vi "Write Functions.vi"(5 "Functions":variant=variant("Absolute Value"=variant(refnum<class "PythonFunction.lvclass"> refnum), "Add"=variant(refnum<class "PythonFunction.lvclass"> refnum), "And"=variant(refnum<class "PythonFunction.lvclass"> refnum), "And Array Elements"=variant(refnum<class "PythonFunction.lvclass"> refnum), "Array Max & Min"=variant(refnum<class "PythonFunction.lvclass"> refnum), "Array Size"=variant(refnum<class "PythonFunction.lvclass"> refnum), "Array Subset"=variant(refnum<class "PythonFunction.lvclass"> refnum), "Array of Strings To Path"=variant(refnum<class "PythonFunction.lvclass"> refnum), "Build Array"=variant(refnum<class "PythonFunction.lvclass"> refnum), "Build Path"=variant(refnum<class "PythonFunction.lvclass"> refnum), "Byte Array To String"=variant(refnum<class "PythonFunction.lvclass"> refnum), "Close File"=variant(refnum<class "PythonFunction.lvclass"> refnum), "Concatenate Strings"=variant(refnum<class "PythonFunction.lvclass"> refnum), "Cosecant"=variant(refnum<class "PythonFunction.lvclass"> refnum), "Cosine"=variant(refnum<class "PythonFunction.lvclass"> refnum), "Cotangent"=variant(refnum<class "PythonFunction.lvclass"> refnum), "Decimal String To Number"=variant(refnum<class "PythonFunction.lvclass"> refnum), "Decimate 1D Array"=variant(refnum<class "PythonFunction.lvclass"> refnum), "Delete From Array"=variant(refnum<class "PythonFunction.lvclass"> refnum), "Divide"=variant(refnum<class "PythonFunction.lvclass"> refnum), "Empty Array?"=variant(refnum<class "PythonFunction.lvclass"> refnum), "Empty String/Path?"=variant(refnum<class "PythonFunction.lvclass"> refnum), "Equal To 0?"=variant(refnum<class "PythonFunction.lvclass"> refnum), "Equal?"=variant(refnum<class "PythonFunction.lvclass"> refnum), "Exclusive Or"=variant(refnum<class "PythonFunction.lvclass"> refnum), "Exponential"=variant(refnum<class "PythonFunction.lvclass"> refnum), "Exponential(Arg)-1"=variant(refnum<class "PythonFunction.lvclass"> refnum), "Format Value"=variant(refnum<class "PythonFunction.lvclass"> refnum), "Fract/Exp String To Number"=variant(refnum<class "PythonFunction.lvclass"> refnum), "Get Date/Time String"=variant(refnum<class "PythonFunction.lvclass"> refnum), "Greater Or Equal To 0?"=variant(refnum<class "PythonFunction.lvclass"> refnum), "Greater Or Equal?"=variant(refnum<class "PythonFunction.lvclass"> refnum), "Greater Than 0?"=variant(refnum<class "PythonFunction.lvclass"> refnum), "Greater?"=variant(refnum<class "PythonFunction.lvclass"> refnum), "Hexadecimal String To Number"=variant(refnum<class "PythonFunction.lvclass"> refnum), "Hyperbolic Cosecant"=variant(refnum<class "PythonFunction.lvclass"> refnum), "Hyperbolic Cosine"=variant(refnum<class "PythonFunction.lvclass"> refnum), "Hyperbolic Cotangent"=variant(refnum<class "PythonFunction.lvclass"> refnum), "Hyperbolic Secant"=variant(refnum<class "PythonFunction.lvclass"> refnum), "Hyperbolic Sine"=variant(refnum<class "PythonFunction.lvclass"> refnum), "Hyperbolic Tangent"=variant(refnum<class "PythonFunction.lvclass"> refnum), "Implies"=variant(refnum<class "PythonFunction.lvclass"> refnum), "In Range and Coerce"=variant(refnum<class "PythonFunction.lvclass"> refnum), "Index Array"=variant(refnum<class "PythonFunction.lvclass"> refnum), "Initialize Array"=variant(refnum<class "PythonFunction.lvclass"> refnum), "Interleave 1D Arrays"=variant(refnum<class "PythonFunction.lvclass"> refnum), "Inverse Cosecant"=variant(refnum<class "PythonFunction.lvclass"> refnum), "Inverse Cosine"=variant(refnum<class "PythonFunction.lvclass"> refnum), "Inverse Cotangent"=variant(refnum<class "PythonFunction.lvclass"> refnum), "Inverse Hyperbolic Cosecant"=variant(refnum<class "PythonFunction.lvclass"> refnum), "Inverse Hyperbolic Cosine"=variant(refnum<class "PythonFunction.lvclass"> refnum), "Inverse Hyperbolic Cotangent"=variant(refnum<class "PythonFunction.lvclass"> refnum), "Inverse Hyperbolic Secant"=variant(refnum<class "PythonFunction.lvclass"> refnum), "Inverse Hyperbolic Sine"=variant(refnum<class "PythonFunction.lvclass"> refnum), "Inverse Hyperbolic Tangent"=variant(refnum<class "PythonFunction.lvclass"> refnum), "Inverse Secant"=variant(refnum<class "PythonFunction.lvclass"> refnum), "Inverse Sine"=variant(refnum<class "PythonFunction.lvclass"> refnum), "Inverse Tangent"=variant(refnum<class "PythonFunction.lvclass"> refnum), "Inverse Tangent (2 Input)"=variant(refnum<class "PythonFunction.lvclass"> refnum), "Less Or Equal To 0?"=variant(refnum<class "PythonFunction.lvclass"> refnum), "Less Or Equal?"=variant(refnum<class "PythonFunction.lvclass"> refnum), "Less Than 0?"=variant(refnum<class "PythonFunction.lvclass"> refnum), "Less?"=variant(refnum<class "PythonFunction.lvclass"> refnum), "Lexical Class"=variant(refnum<class "PythonFunction.lvclass"> refnum), "Logarithm Base 10"=variant(refnum<class "PythonFunction.lvclass"> refnum), "Logarithm Base 2"=variant(refnum<class "PythonFunction.lvclass"> refnum), "Max & Min"=variant(refnum<class "PythonFunction.lvclass"> refnum), "Multiply"=variant(refnum<class "PythonFunction.lvclass"> refnum), "Natural Logarithm"=variant(refnum<class "PythonFunction.lvclass"> refnum), "Negate"=variant(refnum<class "PythonFunction.lvclass"> refnum), "Not"=variant(refnum<class "PythonFunction.lvclass"> refnum), "Not A Number/Path/Refnum?"=variant(refnum<class "PythonFunction.lvclass"> refnum), "Not And"=variant(refnum<class "PythonFunction.lvclass"> refnum), "Not Equal To 0?"=variant(refnum<class "PythonFunction.lvclass"> refnum), "Not Equal?"=variant(refnum<class "PythonFunction.lvclass"> refnum), "Not Exclusive Or"=variant(refnum<class "PythonFunction.lvclass"> refnum), "Not Or"=variant(refnum<class "PythonFunction.lvclass"> refnum), "Number To Boolean Array"=variant(refnum<class "PythonFunction.lvclass"> refnum), "Number To Decimal String"=variant(refnum<class "PythonFunction.lvclass"> refnum), "Number To Exponential String"=variant(refnum<class "PythonFunction.lvclass"> refnum), "Number To Fractional String"=variant(refnum<class "PythonFunction.lvclass"> refnum), "Number To Hexadecimal String"=variant(refnum<class "PythonFunction.lvclass"> refnum), "Number To Octal String"=variant(refnum<class "PythonFunction.lvclass"> refnum), "Octal String To Number"=variant(refnum<class "PythonFunction.lvclass"> refnum), "Open/Create/Replace File"=variant(refnum<class "PythonFunction.lvclass"> refnum), "Or"=variant(refnum<class "PythonFunction.lvclass"> refnum), "Or Array Elements"=variant(refnum<class "PythonFunction.lvclass"> refnum), "Path To String"=variant(refnum<class "PythonFunction.lvclass"> refnum), "Path to Array of Strings"=variant(refnum<class "PythonFunction.lvclass"> refnum), "Power of 2"=variant(refnum<class "PythonFunction.lvclass"> refnum), "Power of X"=variant(refnum<class "PythonFunction.lvclass"> refnum), "Quotient & Remainder"=variant(refnum<class "PythonFunction.lvclass"> refnum), "Random Number (0-1)"=variant(refnum<class "PythonFunction.lvclass"> refnum), "Read from Text File"=variant(refnum<class "PythonFunction.lvclass"> refnum), "Reciprocal"=variant(refnum<class "PythonFunction.lvclass"> refnum), "Replace Array Subset"=variant(refnum<class "PythonFunction.lvclass"> refnum), "Replace Substring"=variant(refnum<class "PythonFunction.lvclass"> refnum), "Reshape Array"=variant(refnum<class "PythonFunction.lvclass"> refnum), "Reverse 1D Array"=variant(refnum<class "PythonFunction.lvclass"> refnum), "Rotate 1D Array"=variant(refnum<class "PythonFunction.lvclass"> refnum), "Round To Nearest"=variant(refnum<class "PythonFunction.lvclass"> refnum), "Round Toward +Infinity"=variant(refnum<class "PythonFunction.lvclass"> refnum), "Round Toward -Infinity"=variant(refnum<class "PythonFunction.lvclass"> refnum), "Search 1D Array"=variant(refnum<class "PythonFunction.lvclass"> refnum), "Secant"=variant(refnum<class "PythonFunction.lvclass"> refnum), "Seconds To Date/Time"=variant(refnum<class "PythonFunction.lvclass"> refnum), "Select"=variant(refnum<class "PythonFunction.lvclass"> refnum), "Sign"=variant(refnum<class "PythonFunction.lvclass"> refnum), "Sinc"=variant(refnum<class "PythonFunction.lvclass"> refnum), "Sine"=variant(refnum<class "PythonFunction.lvclass"> refnum), "Sine & Cosine"=variant(refnum<class "PythonFunction.lvclass"> refnum), "Sort 1D Array"=variant(refnum<class "PythonFunction.lvclass"> refnum), "Split 1D Array"=variant(refnum<class "PythonFunction.lvclass"> refnum), "Square"=variant(refnum<class "PythonFunction.lvclass"> refnum), "Square Root"=variant(refnum<class "PythonFunction.lvclass"> refnum), "String Length"=variant(refnum<class "PythonFunction.lvclass"> refnum), "String Subset"=variant(refnum<class "PythonFunction.lvclass"> refnum), "String To Byte Array"=variant(refnum<class "PythonFunction.lvclass"> refnum), "String To Path"=variant(refnum<class "PythonFunction.lvclass"> refnum), "Strip Path"=variant(refnum<class "PythonFunction.lvclass"> refnum), "Subtract"=variant(refnum<class "PythonFunction.lvclass"> refnum), "Tangent"=variant(refnum<class "PythonFunction.lvclass"> refnum), "Tick Count (ms)"=variant(refnum<class "PythonFunction.lvclass"> refnum), "To Lower Case"=variant(refnum<class "PythonFunction.lvclass"> refnum), "To Upper Case"=variant(refnum<class "PythonFunction.lvclass"> refnum), "Transpose 2D Array"=variant(refnum<class "PythonFunction.lvclass"> refnum), "Trim Whitespace"=variant(refnum<class "PythonFunction.lvclass"> refnum), "Wait (ms)"=variant(refnum<class "PythonFunction.lvclass"> refnum), "Wait Until Next ms Multiple"=variant(refnum<class "PythonFunction.lvclass"> refnum)), 9 "PythonConverter_BD in":refnum<class "PythonBDConverter.lvclass">) -> (3 "PythonConverter_BD out":refnum<class "PythonBDConverter.lvclass">)   [LabVIEW 2014, in "PythonBDConverter.lvclass"]
uses:
  PythonBDConverter.lvclass
  Parsing/Classes/PythonFunction/PythonFunction.lvclass
  PythonBDConverter.lvclass/PythonBDConverter.ctl
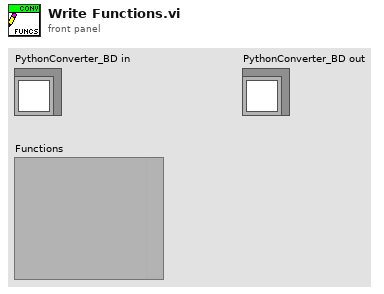
[diagram p1: front panel]
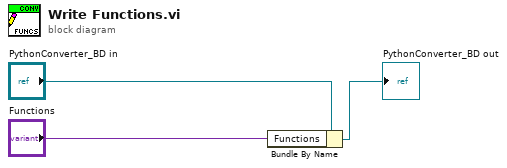
[diagram p0: block diagram]
diagram:
  n1 = Bundle By Name(cluster="PythonConverter_BD in", "Functions"="Functions") -> (→"PythonConverter_BD out":refnum<class "PythonBDConverter.lvclass">)
